vi "DAQmx Start Trigger (Digital Pattern).vi"(0 "task/channels in":refnum<k21>, 1 "trigger when":i32(ring)=10254 items=["Pattern Matches"=10254, "Pattern Does Not Match"=10253], 5 "source":tag, 7 "pattern":string, 11 "error in":errorcluster) -> (4 "task out":refnum<k21>, 15 "error out":errorcluster)   [LabVIEW 2011]
doc: "Configures a task to start acquiring or generating samples when a digital pattern is matched."
uses:
  C:/Program Files/National Instruments/LabVIEW 2011/resource/objmgr/daqmx.rc
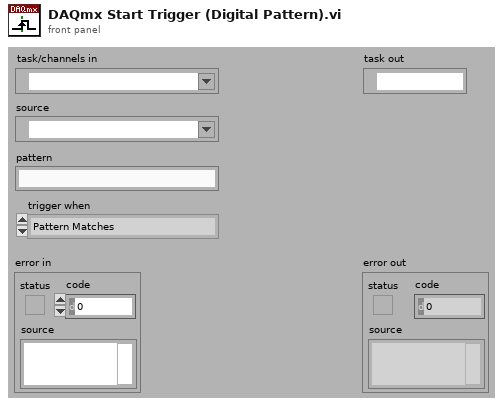
[diagram p1: front panel]
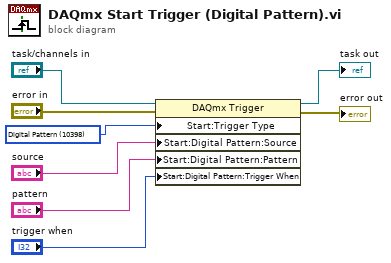
[diagram p0: block diagram]
diagram:
  w4 = 10398 items=["Analog Edge"=10099, "Digital Edge"=10150, "Analog Window"=10103, "Digital Pattern"=10398, "None"=10230] ("Start.TrigType")
  n1 = property class="DAQmx Trigger"(reference="task/channels in", error in="error in", "Start:Trigger Type"=w4, "Start:Digital Pattern:Source"="source", "Start:Digital Pattern:Pattern"="pattern", "Start:Digital Pattern:Trigger When"="trigger when") -> (reference out=→"task out":refnum<k21>, error out=→"error out":errorcluster)
